vi "String to String Array.vi"(11 "String":string) -> (3 "Array":string[][](array[string]))   [LabVIEW 2019, in "Muon Data Post-Processing.lvlib"]
uses:
  Muon Data Post-Processing.lvlib
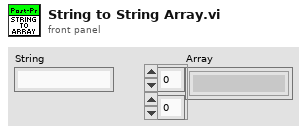
[diagram p1: front panel]
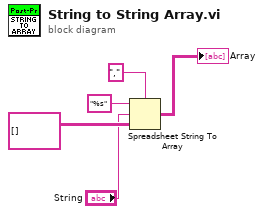
[diagram p0: block diagram]
diagram:
  n1 = Spreadsheet String To Array(delimiter (Tab)=",", format string="%s", spreadsheet string="String", array type (2D Dbl)=string[][] []) -> (array=→"Array":string[][])
